vi "stop_sweep.vi"(8 "error in (no error)":errorcluster, 11 "DL090130ExperimentController in":refnum<class "ExperimentControllerDL090130Interval.lvclass">) -> (0 "error out":errorcluster, 3 "DL090130ExperimentController out":refnum<class "ExperimentControllerDL090130Interval.lvclass">)   [LabVIEW 2010, in "ExperimentControllerDL090130Interval.lvclass"]
uses:
  ExperimentControllerDL090130Interval.lvclass
  common/classes/ErrorController/ErrorController/class_data.vi
  ImagingMode/GenericImagingMode/GenericImagingMode/GenericImagingMode.lvclass
  common/classes/ErrorController/ErrorController/ErrorController.lvclass
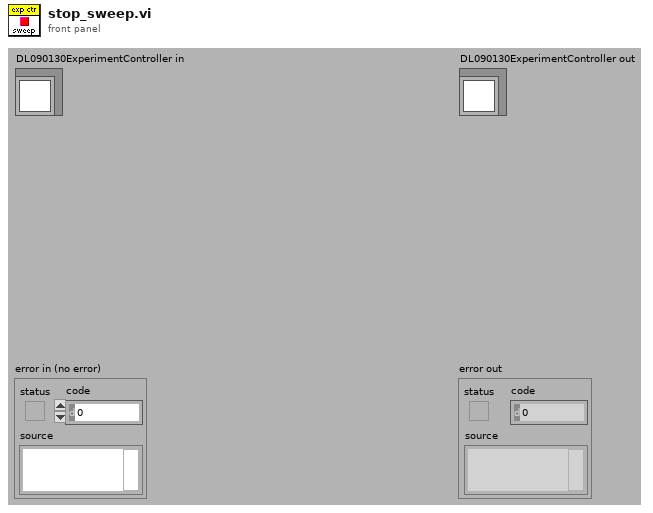
[diagram p1: front panel]
types:
  T1 = typedef "GenericToplevelComponent.lvclass/common_trigger_enum.ctl" = enum16{"NULL", "initialise", "terminate", "fetch command", "fetch data", "attach observer", "register as observer", "detach observer", "acknowledge", "start", "stop", "sweep started", "sweep finished", "experiment started", "experiment stopped"}
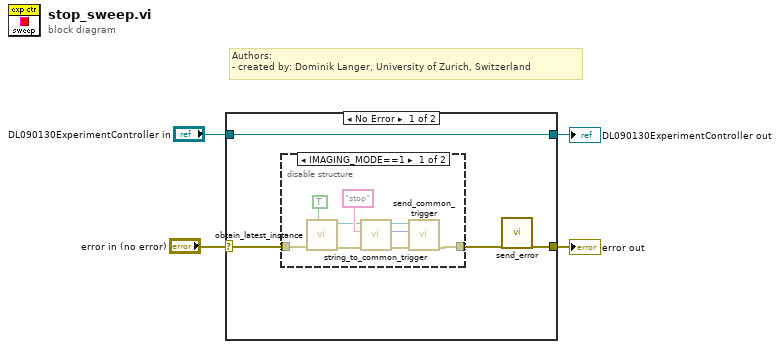
[diagram p0: block diagram]
diagram:
  # "Authors: \n- created by: Dominik Langer, University of Zurich, Switzerland"
  n1 = case shown="No Error" "error in (no error)" {
    selector: "error in (no error)" -> [w7 w20]
    tunnel: [w6 w20] -> w3
    tunnel: [w8 w19] -> w1
    tunnel: "DL090130ExperimentController in" -> [w8 w19]
    frame No Error {
      n2 = disable-structure shown="IMAGING_MODE==1" {
        disable-tunnel: w7 -> [w17 w18]
        disable-tunnel: [w16 w18] -> w5
        frame condition #0 {
          n3 = call "obtain_latest_instance.vi"("quick, but maybe outdated?"=TRUE, "error in (no error)"=w17) -> ("error out"=w13:errorcluster, "GenericScanMode out"=w11:refnum<class "GenericImagingMode.lvclass">)  [unwired: 8 in]
          n4 = call-dynamic "string_to_common_trigger.vi"("error in (no error)"=w13, "trigger string"="stop", "GenericToplevelComponent in"=w11) -> ("error out"=w12:errorcluster, "trigger"=w9:T1, "GenericToplevelComponent out"=w10:refnum<class "GenericImagingMode.lvclass">)  [unwired: 6 in]
          n5 = call-dynamic "send_common_trigger.vi"("error in (no error)"=w12, "trigger"=w9, "GenericToplevelComponent in"=w10) -> ("error out"=w16:errorcluster)  [unwired: 6 in, 2 out]
        }
        frame condition #1 (active) {
        }
      }
      n6 = call "send_error.vi"("error in (no error)"=w5) -> ("error out"=w6:errorcluster)  [unwired: 10 in]
    }
    frame Error {
    }
  }
  "error out" <- w3
  "DL090130ExperimentController out" <- w1
